vi "LS218_DETECTION_PORT_COM.vi"(8 "error in (no error)":errorcluster caption="entrée d'erreur (pas d'erreur)", 10 "baud rate (9600)":u32=9600 caption="débit en bauds (9600)") -> (0 "sortie d'erreur":errorcluster, 1 "Port trouvé?":bool, 2 "Réponse IDN":string, 3 "Nom de ressource VISA en sortie":refnum<visa-resource-name>)   [LabVIEW 2014]
uses:
  <vilib>/Instr/_visa.llb/VISA Find Search Mode.ctl
  <vilib>/Instr/_visa.llb/VISA Set IO Buffer Mask.ctl
  <vilib>/Instr/_visa.llb/VISA Flush IO Buffer Mask.ctl
  <vilib>/Instr/_visa.llb/VISA Configure Serial Port (Instr).vi
panel:
  out "liste trouvée":string[](array[string])
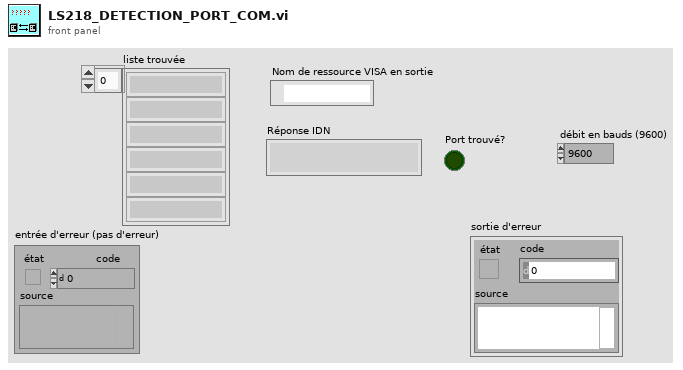
[diagram p1: front panel]
types:
  T1 = typedef "VISA Find Search Mode.ctl" = u32
  T2 = typedef "VISA Flush IO Buffer Mask.ctl" = u16
  T3 = typedef "VISA Set IO Buffer Mask.ctl" = u16
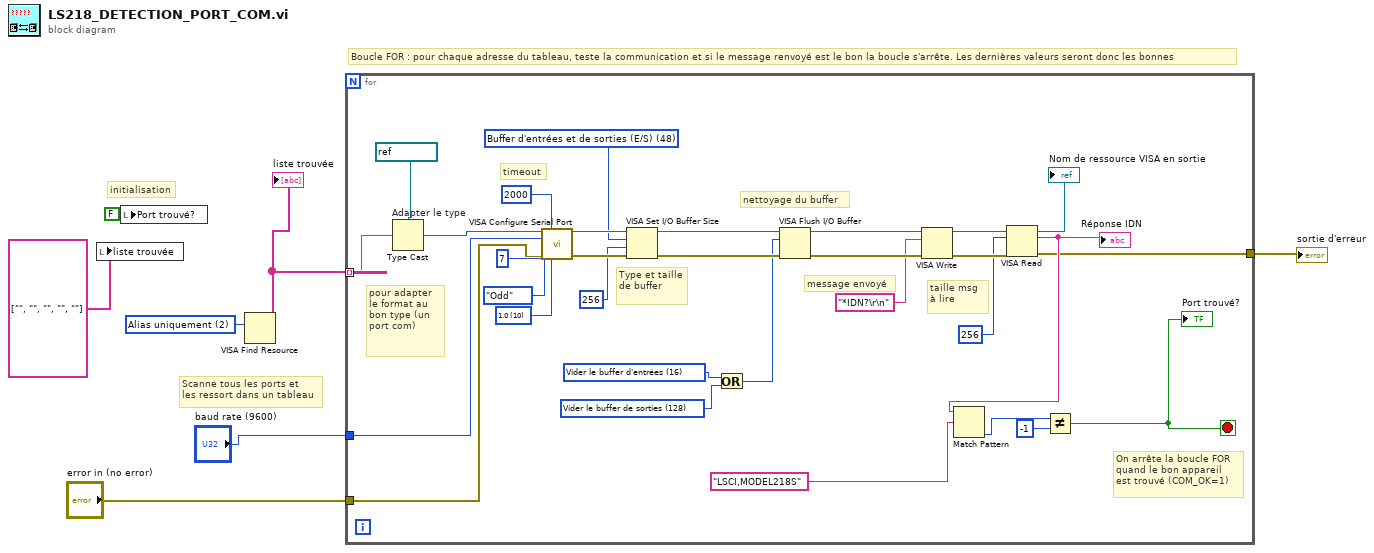
[diagram p0: block diagram]
diagram:
  w7 = T1 2 items=["Noms canoniques uniquement"=0, "Alias uniquement"=2, "Inclure les alias correspondants"=3, "Inclure tous les alias"=4] ("Search Mode")
  # "initialisation"
  # "Scanne tous les ports et\nles ressort dans un tableau"
  # "Boucle FOR : pour chaque adresse du tableau, teste la communication et si le message renvoyé est le bon la boucle s'arrête. Les dernières valeurs seront donc les bonnes"
  n1 = local write "liste trouvée"(string[] ["", "", "", "", ""] ("liste trouvée")) -> ()
  n2 = local write "Port trouvé?"(FALSE ("COM_OK")) -> ()
  n3 = VISA Find Resource(10:w7) -> (3:w6:string[])  [unwired: 2 in, 2 out]
  "liste trouvée" <- w6
  n4 = for {
    tunnel: w6 -> [w22] mode=indexing
    tunnel: [w10] -> w3
    tunnel: "baud rate (9600)" -> [w9]
    tunnel: "error in (no error)" -> [w8]
    stop <- w15 stop-if-true
    w11 = u16 10 items=["1.0"=10, "1.5"=15, "2.0"=20] ("stop bits (10: 1 bit)")
    w30 = T2 128 items=["Vider le buffer d'entrées"=16, "Écrire le buffer de sorties sur le périphérique"=32, "Vider le buffer d'entrées (Pas d'E/S)"=64, "Vider le buffer de sorties"=128] ("Mask")
    w31 = T2 16 items=["Vider le buffer d'entrées"=16, "Écrire le buffer de sorties sur le périphérique"=32, "Vider le buffer d'entrées (Pas d'E/S)"=64, "Vider le buffer de sorties"=128] ("Mask")
    w34 = T3 48 items=["Buffer d'entrées (E/S)"=16, "Buffer de sorties (E/S)"=32, "Buffer d'entrées et de sorties (E/S)"=48] ("Mask")
    # "timeout"
    # "On arrête la boucle FOR\nquand le bon appareil\nest trouvé (COM_OK=1)"
    # "pour adapter\nle format au \nbon type (un port com)"
    # "taille msg à lire"
    # "message envoyé"
    # "nettoyage du buffer"
    # "Type et taille de buffer"
    n5 = Type Cast "Adapter le type"(type=refnum<visa-resource-name> "COM1" ("VISA resource name"), x=w22) -> (*(type *) &x=w21:refnum<visa-resource-name>)
    n6 = call-poly "VISA Configure Serial Port"("VISA resource name"=w21, "timeout (10sec)"=u32 2000, "baud rate (9600)"=w9, "data bits (8)"=u16 7, "parity (0:none)"=enum16{"None", "Odd", "Even", "Mark", "Space"}."Odd", "error in (no error)"=w8, "stop bits (10: 1 bit)"=w11) -> ("VISA resource name out"=w37:refnum<visa-resource-name>, "error out"=w36:errorcluster)  [unwired: 7 in]
    n7 = VISA Set I/O Buffer Size(VISA resource name=w37, mask (16)=w34, size (4096)=u32 256 ("taille (4096)"), error in (no error)=w36) -> (VISA resource name out=w32:refnum<visa-resource-name>, error out=w33:errorcluster)
    n8 = Or(x=w31, y=w30) -> (x .or. y?=w29:T2)
    n9 = VISA Flush I/O Buffer(VISA resource name=w32, mask (16)=w29, error in (no error)=w33) -> (VISA resource name out=w27:refnum<visa-resource-name>, error out=w28:errorcluster)
    n10 = VISA Write(VISA resource name=w27, write buffer="*IDN?\r\n" ("buffer d'écriture"), error in (no error)=w28) -> (VISA resource name out=w24:refnum<visa-resource-name>, error out=w25:errorcluster)  [unwired: 1 out]
    "Nom de ressource VISA en sortie" <- w24
    n11 = VISA Read(VISA resource name=w24, byte count=u32 256 ("nombre d'octets"), error in (no error)=w25) -> (read buffer=w14:string, error out=w10:errorcluster)  [unwired: 2 out]
    "Réponse IDN" <- w14
    n12 = Match Pattern(string=w14, regular expression="LSCI,MODEL218S" ("y")) -> (offset past match=w17:i32)  [unwired: 1 in, 3 out]
    n13 = Not Equal?(x=w17, y=-1) -> (x != y?=w15:bool)
    "Port trouvé?" <- w15
  }
  "sortie d'erreur" <- w3
